vi "Acquisition Params.vi"() -> ()   [LabVIEW 2020]
uses:
  Acquisition Params.ctl
panel:
  in  "Acquisition Params":T1 {"Interval" min=0.0 max=99999.0; "Frames" min=0.0 max=5000.0; "ExposureMs" min=0.0 max=99999.0}
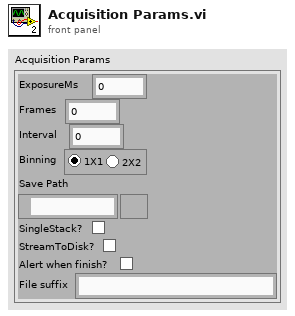
[diagram p1: front panel]
types:
  T1 = typedef "Acquisition Params.ctl" = cluster{"ExposureMs":dbl, "Frames":dbl, "Interval":dbl, "Binning":enum32{"1x1", "2x2"}, "Save Path":path, "SingleStack?":bool, "StreamToDisk?":bool, "Alert when finish?":bool, "File suffix":string}
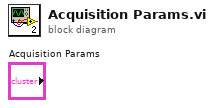
[diagram p0: block diagram]
diagram:
